vi "Get SMO Port.vi"(8 "error in (no error)":errorcluster, 11 "Inst.Xeryon-RotatorInstrument in":refnum<class "Inst.Xeryon-Rotator.lvclass">) -> (0 "error out":errorcluster, 2 "Port":u16, 3 "Inst.Xeryon-RotatorInstrument out":refnum<class "Inst.Xeryon-Rotator.lvclass">)   [LabVIEW 2019, in "Inst.Xeryon-Rotator.lvclass"]
uses:
  Inst.Xeryon-Rotator.lvclass
  <userlib>/LevyLab/Instrument Framework/Instrument Types/Cryostat/Instrument.Cryostat.lvclass
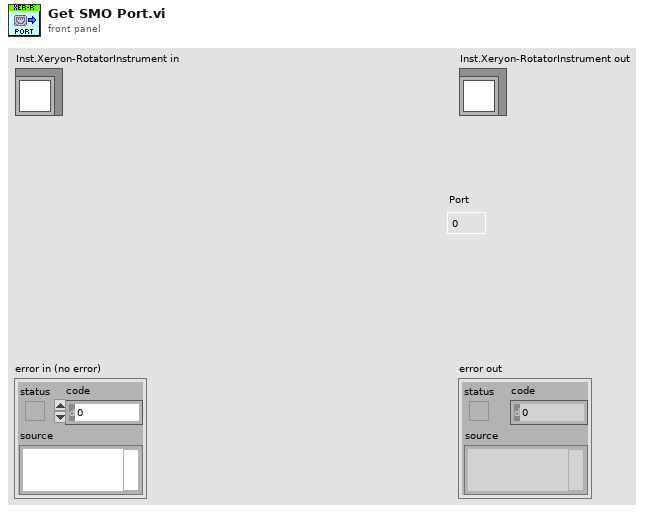
[diagram p1: front panel]
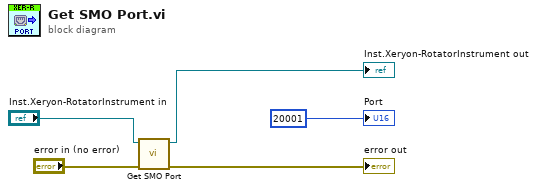
[diagram p0: block diagram]
diagram:
  n1 = call-parent "Get SMO Port.vi"("error in (no error)"="error in (no error)", "Instrument in"="Inst.Xeryon-RotatorInstrument in") -> ("error out"=→"error out":errorcluster, "Instrument out"=→"Inst.Xeryon-RotatorInstrument out":refnum<class "Inst.Xeryon-Rotator.lvclass">)  [unwired: 7 in, 1 out]
  "Port" <- u16 20001 ("Port")
